vi "Initialize.vi"(8 "error in (no error)":errorcluster, 10 "Transfer Configuration":T1 {"channel configurations"."buffer offset" format="%d bytes"}, 11 "Transfer Configuration type":refnum<class "Transfer Configuration.lvclass">) -> (0 "error out":errorcluster, 3 "Transfer Configuration out":refnum<class "Transfer Configuration.lvclass">)   [LabVIEW 2017, in "DSF Core.lvlib" / "Transfer Configuration.lvclass"]
uses:
  Transfer Configuration.lvclass
  Configuration.lvclass
  C:/Git/DSF/Data Sharing Framework/Source/Core/Engine/Classes/Configuration/Configuration.lvclass
  DSF Configuration API/Public/Controls/DSF Byte Order.ctl
  DSF Core.lvlib
  DSF Configuration API/Public/Controls/DSF Data Type.ctl
  DSF Configuration API/Public/Controls/DSF Engine Channel Configuration.ctl
  DSF Configuration API/Public/Controls/DSF Settings Info.ctl
  DSF Configuration API/Public/Controls/DSF Engine Transfer Configuration.ctl
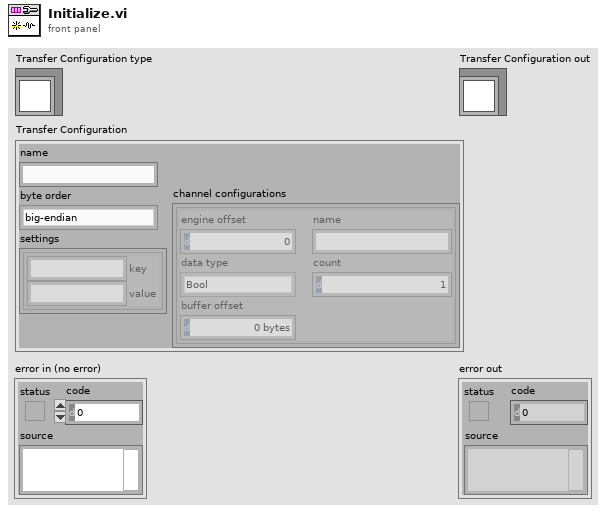
[diagram p1: front panel]
types:
  T1 = typedef "DSF Core.lvlib/DSF Engine Transfer Configuration.ctl" = cluster{"name":string, "byte order":T2, "channel configurations":T3[], "settings":T5}
  T2 = typedef "DSF Core.lvlib/DSF Byte Order.ctl" = enum8{"big-endian", "little-endian"}
  T3 = typedef "DSF Core.lvlib/DSF Engine Channel Configuration.ctl" = cluster{"engine offset":u64, "name":string, "data type":T4, "count":u64, "buffer offset":u64}
  T4 = typedef "DSF Core.lvlib/DSF Data Type.ctl" = enum8{"Bool", "SGL", "DBL", "I8", "I16", "I32", "I64", "U8", "U16", "U32", "U64"}
  T5 = typedef "DSF Core.lvlib/DSF Settings Info.ctl" = cluster{"key":string, "value":string}[]
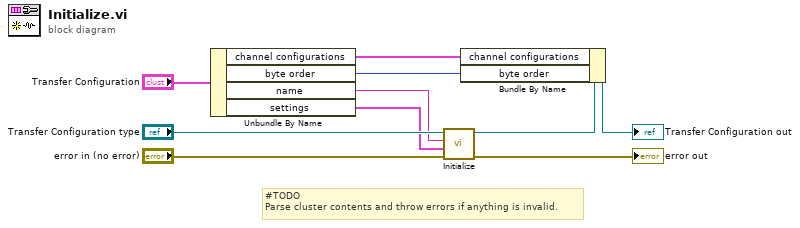
[diagram p0: block diagram]
diagram:
  # "#TODO\nParse cluster contents and throw errors if anything is invalid."
  n1 = Unbundle By Name("Transfer Configuration") -> ("channel configurations"=w2:T3[], "byte order"=w1:T2, "name"=w3:string, "settings"=w4:T5)
  n2 = call "Initialize.vi"("error in (no error)"="error in (no error)", "settings"=w4, "name"=w3, "Configuration in"="Transfer Configuration type") -> ("error out"=→"error out":errorcluster, "Configuration out"=w8:refnum<class "Transfer Configuration.lvclass">)  [unwired: 6 in]
  n3 = Bundle By Name(cluster=w8, "channel configurations"=w2, "byte order"=w1) -> (→"Transfer Configuration out":refnum<class "Transfer Configuration.lvclass">)
